vi "conductivitysensor.vi"() -> ()   [LabVIEW 2023]
uses:
  <vilib>/Instr/_visa.llb/VISA Configure Serial Port (Instr).vi
panel:
  out "match + rest of string":string
  in  "search string/char (-)":string
  out "read buffer":string
  out "return count":u32
  out "error out":errorcluster
  out "?":u32
  in  "VISA resource name":refnum<visa-resource-name>
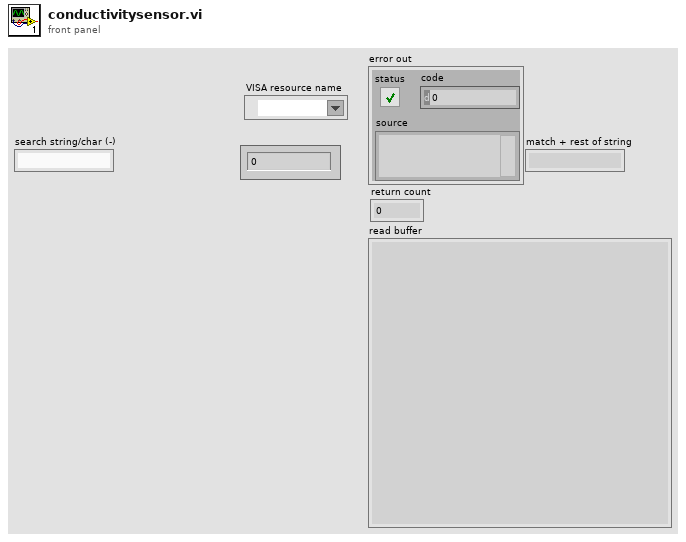
[diagram p1: front panel]
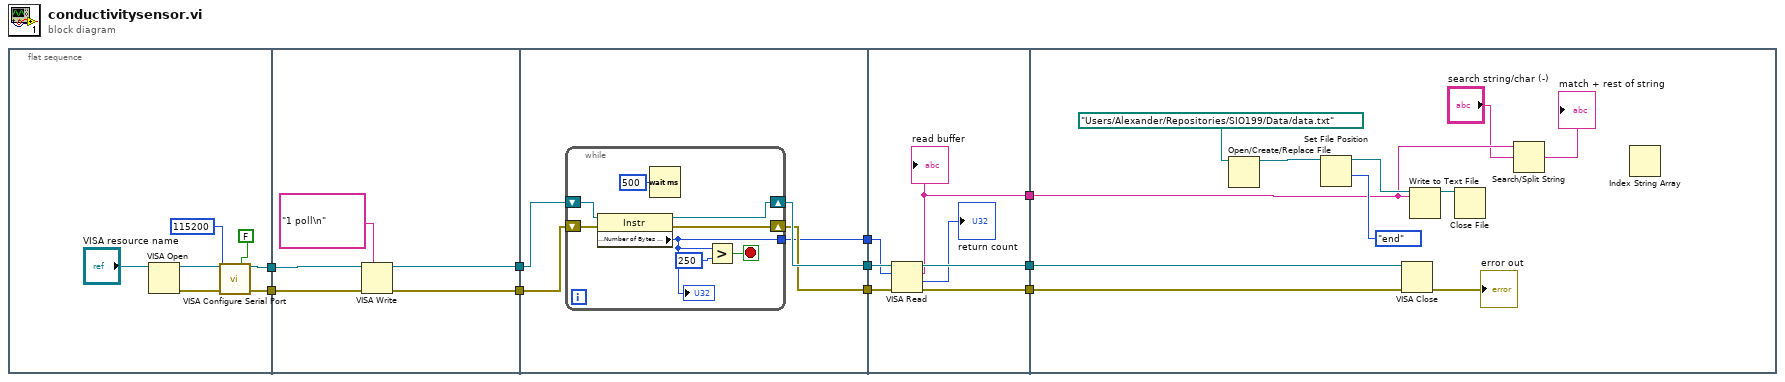
[diagram p0: block diagram]
diagram:
  n1 = flat-sequence {
    tunnel: [w16] -> w9
    tunnel: [w14] -> w3
    tunnel: [w22] -> w8
    tunnel: w9 -> [w21]
    tunnel: [w20] -> w4
    tunnel: w3 -> [w19]
    tunnel: w8 -> [w27]
    tunnel: [w26] -> w7
    tunnel: [w25] -> w5
    tunnel: w4 -> [w24]
    tunnel: [w23] -> w2
    tunnel: [w42] -> w10
    tunnel: w7 -> [w41]
    tunnel: [w40] -> w6
    tunnel: w5 -> [w39]
    tunnel: w2 -> [w38]
    tunnel: [w36] -> w1
    tunnel: w10 -> [w53]
    tunnel: w6 -> [w52]
    tunnel: w1 -> [w45]
    frame #0 {
      n2 = VISA Open(VISA resource name="VISA resource name") -> (VISA resource name=w15:refnum<visa-resource-name>, error out=w13:errorcluster)  [unwired: 4 in]
      n3 = call-poly "VISA Configure Serial Port"("VISA resource name"=w15, "Enable Termination\nChar (T)"=FALSE, "baud rate (9600)"=u32 115200, "error in (no error)"=w13) -> ("VISA resource name out"=w16:refnum<visa-resource-name>, "error out"=w14:errorcluster)  [unwired: 10 in]
    }
    frame #1 {
      n4 = VISA Write(VISA resource name=w21, write buffer="1 poll\n", error in (no error)=w19) -> (VISA resource name out=w22:refnum<visa-resource-name>, error out=w20:errorcluster)  [unwired: 1 out]
    }
    frame #2 {
      n5 = while {
        tunnel: [w30] -> w23
        shift-right: [w33] -> w25
        shift-left: w24 -> [w28]
        shift-right: [w34] -> w26
        shift-left: w27 -> [w29]
        stop <- w31 stop-if-true
        n6 = property class="Instr"(reference=w29, error in=w28) -> (reference out=w34:refnum<visa-resource-name>, error out=w33:errorcluster, "Serial Settings:Number of Bytes at Serial Port"=w30:u32)
        "?" <- w30
        n7 = Wait (ms)(milliseconds to wait=500) -> ()  [unwired: 1 out]
        n8 = Greater?(x=w30, y=u32 250 ("Serial Settings:Number of Bytes at Serial Port")) -> (0:w31:bool)
      }
    }
    frame #3 {
      n9 = VISA Read(VISA resource name=w41, byte count=w38, error in (no error)=w39) -> (VISA resource name out=w42:refnum<visa-resource-name>, read buffer=w36:string, return count=→"return count":u32, error out=w40:errorcluster)
      "read buffer" <- w36
    }
    frame #4 {
      n10 = Open/Create/Replace File(file path (use dialog)=path "/Users/Alexander/Repositories/SIO199/Data/data.txt") -> (refnum out=w48:refnum<file>)  [unwired: 5 in, 2 out]
      n11 = Set File Position(refnum=w48, from (0:start)=enum16{"start", "end", "current"}."end") -> (refnum out=w49:refnum<file>)  [unwired: 2 in, 1 out]
      n12 = VISA Close(VISA resource name=w53, error in (no error)=w52) -> (error out=→"error out":errorcluster)
      n13 = Write to Text File(file (use dialog)=w49, text=w45) -> (refnum out=w46:refnum<file>)  [unwired: 2 in, 2 out]
      n14 = Close File(refnum=w46) -> ()  [unwired: 1 in, 2 out]
      n15 = Search/Split String(string=w45, search string/char (-)="search string/char (-)") -> (match + rest of string=→"match + rest of string":string)  [unwired: 1 in, 2 out]
      n16 = Index String Array() -> ()  [unwired: 3 in, 1 out]
    }
  }
